vi "Puff_using_Arduino_oneshot.vi"(0 "Puff_duration:Sec":dbl=1.0 format="%.2g") -> ()   [LabVIEW 2022 SP3]
uses:
  Globals/Meas_global.vi
  Controls/Post_Process.ctl
  Controls/Setup.ctl
  Globals/Dynamic_call_global.ph.vi
panel:
  out "Puff Time used":dbl=1.0 format="%.2g"
  out "Case Currently On":string="Loop"
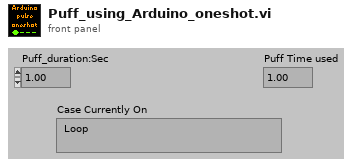
[diagram p1: front panel]
types:
  T1 = typedef "Setup.ctl" = enum16{"Run Program", "Show Setup", "Save Current Setup", "Setup Front Panel"}
  T2 = typedef "Post_Process.ctl" = enum16{"Take New Data", "Post Process Raw Data File"}
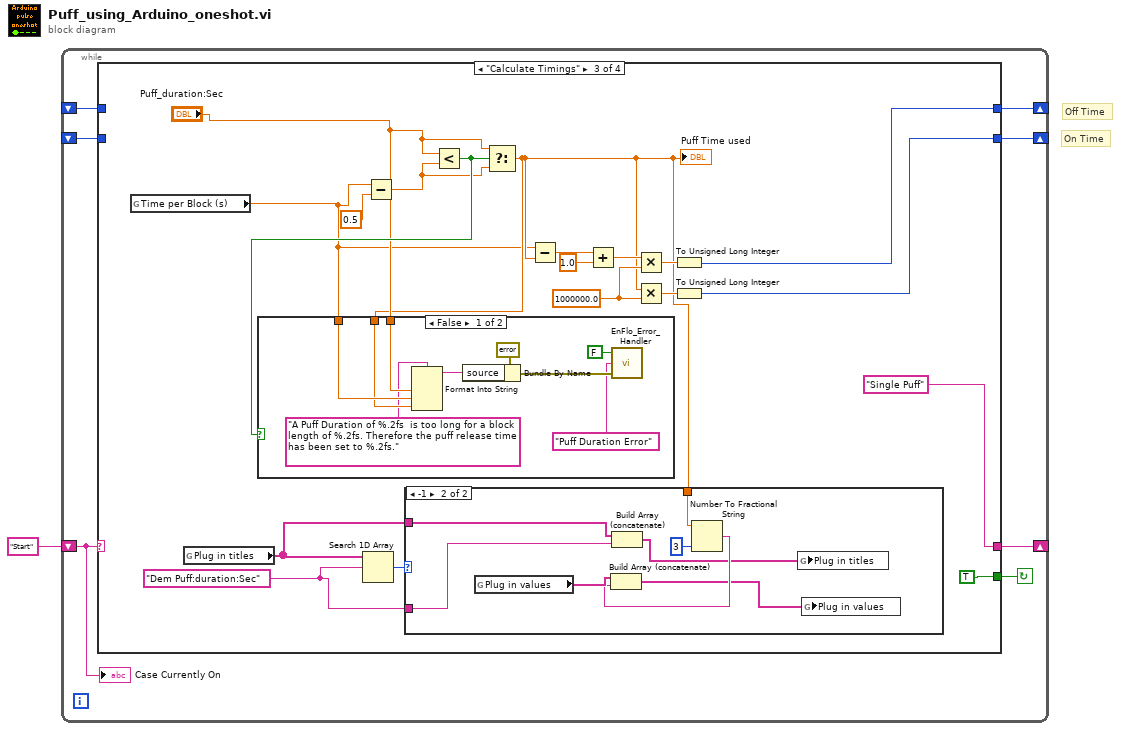
[diagram p0: block diagram]
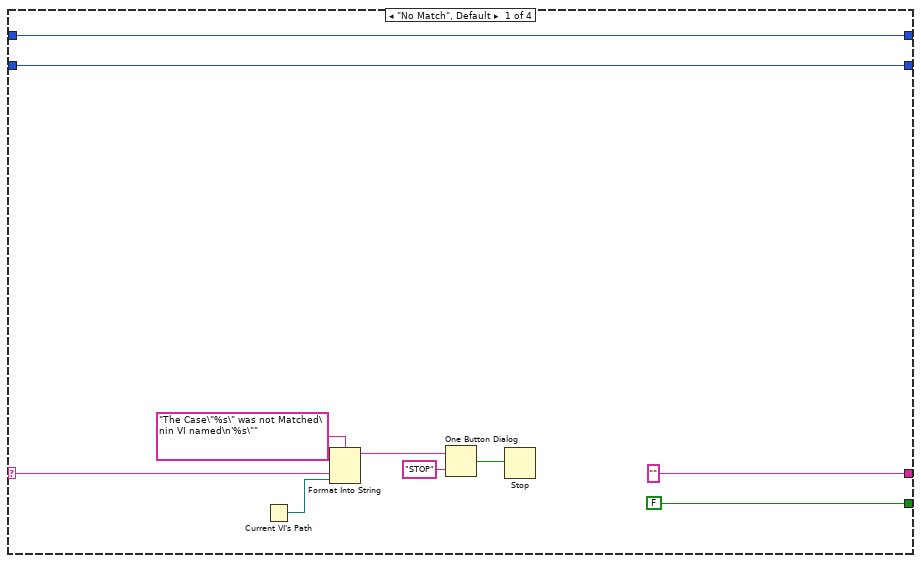
[diagram p2: hidden frame]
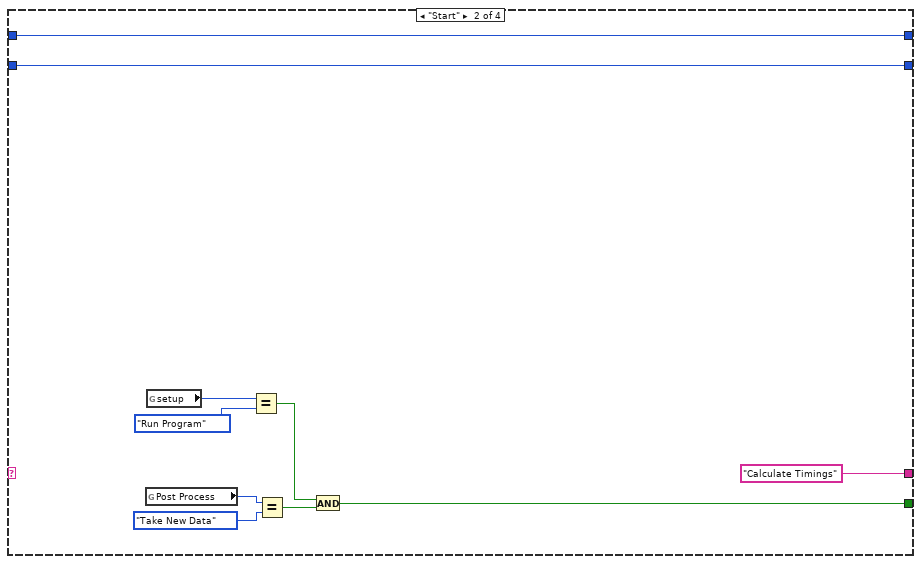
[diagram p3: hidden frame]
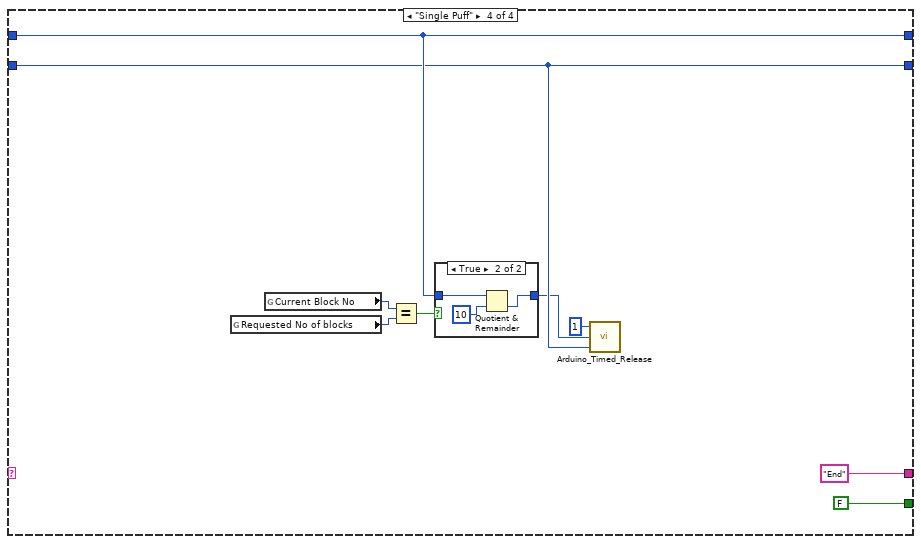
[diagram p6: hidden frame]
diagram:
  # "On Time"
  # "Off Time"
  n1 = while {
    shift-left: "Start" -> [w6]
    shift-right: [w7] -> _
    shift-right: [w5] -> _
    shift-left: _ -> [w4]
    shift-right: [w3] -> _
    shift-left: _ -> [w2]
    stop <- w8 continue-if-true
    n2 = case shown="\"Calculate Timings\"" w6 {
      selector: w6 -> [w9 _ _ _]
      tunnel: [FALSE w21 TRUE ("Command Found") FALSE ("Command Found")] -> w8
      tunnel: ["" "Calculate Timings" "Single Puff" "End"] -> w7
      tunnel: [w11 w20 w38 w73] -> w5
      tunnel: w4 -> [w11 w20 _ w73]
      tunnel: [w10 w19 w37 w72] -> w3
      tunnel: w2 -> [w10 w19 _ w72]
      frame "No Match", Default {
        n3 = Current VI's Path() -> (path=w13:path)
        n4 = Format Into String(format string="The Case\"%s\" was not Matched\nin VI named\n'%s\"" ("Format String"), w9, w13) -> (resulting string=w16:string)  [unwired: 2 in, 1 out]
        n5 = One Button Dialog(message=w16, button name ("OK")="STOP") -> (true=w14:bool)
        n6 = Stop(stop? (T)=w14) -> ()
      }
      frame "Start" {
        n7 = global read "Meas_global.vi" "Post Process"() -> (w23:T2)
        n8 = global read "Meas_global.vi" "setup"() -> (w22:T1)
        n9 = Equal?(x=w22, y=Setup."Run Program") -> (x = y?=w27:bool)
        n10 = Equal?(x=w23, y=Post_Process."Take New Data" ("Post Process")) -> (x = y?=w26:bool)
        n11 = And(x=w27, y=w26) -> (x .and. y?=w21:bool)
      }
      frame "Calculate Timings" {
        w33 = "Dem Puff:duration:Sec"
        w43 = 1000000.0 ("y")
        n12 = global read "Meas_global.vi" "Time per Block (s)"() -> (w31:dbl)
        n13 = global read "Dynamic_call_global.ph.vi" "Plug in titles"() -> (w34:string[])
        n14 = Search 1D Array(1D array=w34, element=w33) -> (index of element=w35:i32)  [unwired: 1 in]
        n15 = Subtract(x=w31, y=0.5) -> (x-y=w29:dbl)
        n16 = Less?(x="Puff_duration:Sec", y=w29) -> (x < y?=w39:bool)
        n17 = Select(t="Puff_duration:Sec", s=w39, f=w29) -> (s? t:f=w32:dbl)
        "Puff Time used" <- w32
        n18 = case shown="False" w39 {
          tunnel: "Puff_duration:Sec" -> [w62 _]
          tunnel: w31 -> [w61 _]
          tunnel: w32 -> [w60 _]
          frame False {
            n19 = Format Into String(format string="A Puff Duration of %.2fs  is too long for a block length of %.2fs. Therefore the puff release time has been set to %.2fs.", w62, w61, w60) -> (resulting string=w58:string)  [unwired: 2 in, 1 out]
            n20 = Bundle By Name(cluster=errorcluster {"status"=TRUE, "code"=0, "source"=""} ("error in (no error)"), "source"=w58) -> (w63:errorcluster)
            n21 = call "EnFlo_Error_Handler.vi"("error in (no error)"=w63, "Error Type"="Puff Duration Error", "Dialog Box (F)"=FALSE ("Dialog Box (T)")) -> ()  [unwired: 1 in, 2 out]
          }
          frame True {
          }
        }
        n22 = case shown="-1" w35 {
          tunnel: w34 -> [_ w54]
          tunnel: w33 -> [_ w53]
          tunnel: w32 -> [_ w52]
          frame Default {
          }
          frame -1 {
            n23 = global read "Dynamic_call_global.ph.vi" "Plug in values"() -> (w55:string[])
            n24 = Build Array (concatenate)(w54, w53) -> (w48:string[])
            n25 = Number To Fractional String(number=w52, precision (6)=i16 3) -> (F-format string=w50:string)  [unwired: 2 in]
            n26 = Build Array (concatenate)(w55, w50) -> (w49:string[])
            n27 = global write "Dynamic_call_global.ph.vi" "Plug in titles"(w48) -> ()
            n28 = global write "Dynamic_call_global.ph.vi" "Plug in values"(w49) -> ()
          }
        }
        n29 = Subtract(x=w31, y=w32) -> (x-y=w42:dbl)
        n30 = Add(x=w42, y=1.0) -> (x+y=w40:dbl)
        n31 = Multiply(x=w40, y=w43) -> (x*y=w44:dbl)
        n32 = Multiply(x=w32, y=w43) -> (x*y=w45:dbl)
        n33 = To Unsigned Long Integer(number=w44) -> (unsigned 32bit integer=w38:u32)
        n34 = To Unsigned Long Integer(number=w45) -> (unsigned 32bit integer=w37:u32)
      }
      frame "Single Puff" {
        n35 = global read "Meas_global.vi" "Requested No of blocks"() -> (w67:i32)
        n36 = global read "Meas_global.vi" "Current Block No"() -> (w66:i32)
        n37 = Equal?(x=w66, y=w67) -> (x = y?=w65:bool)
        n38 = case shown="True" w65 {
          tunnel: w73 -> [w74 w77]
          tunnel: [w74 w75] -> w68
          frame False {
          }
          frame True {
            n39 = Quotient & Remainder(x=w77, y=u32 10) -> (floor(x/y)=w75:u32)  [unwired: 1 out]
          }
        }
        n40 = call "Arduino_Timed_Release.vi"("Time to hold source ON (microseconds)"=w72, "Time to hold source OFF (microseconds)"=w68, "Number of cycles"=u16 1) -> ()  [unwired: 2 out]
      }
    }
    "Case Currently On" <- w6
  }
